vi "HTTPMethod_1.vi"(7 "LabVIEW Web Service Request":refnum<class "Web Request.lvclass">) -> ()   [LabVIEW 2021]
uses:
  <vilib>/wsapi/Web Request.lvclass
panel:
  out "request variables":cluster{"Key":string[], "Value":string[]}
  out "postdata":string
  out "value":string[](array[string])
  # "Use the Web Service Request input terminal to call the VIs on the Web Services palette. Do not remove it from the connector pane unless you don't need access to the palette."
  # "Each additional control wired to the connector pane will be available as an input in the URL. To include an indicator in terminal-mode output (the default setting), it must also be wired to the connector pane."
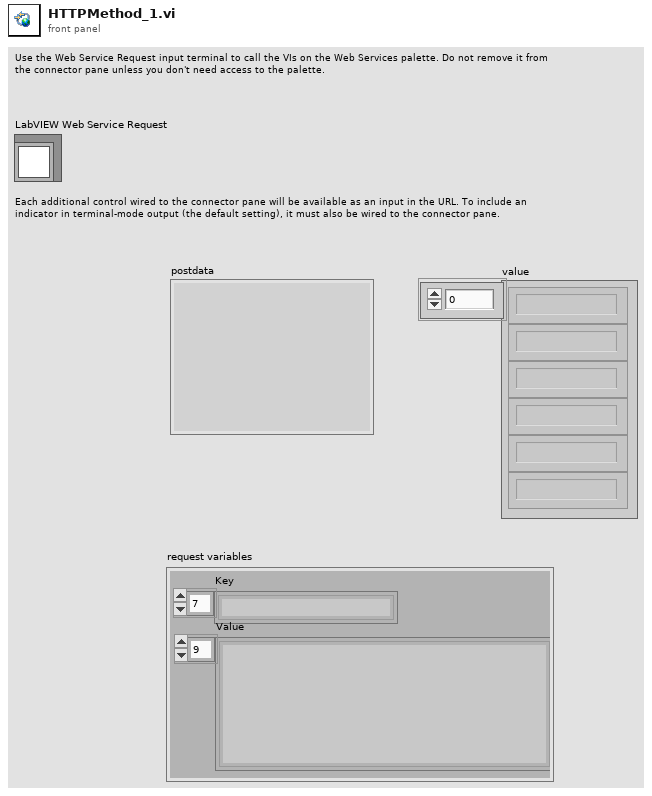
[diagram p1: front panel]
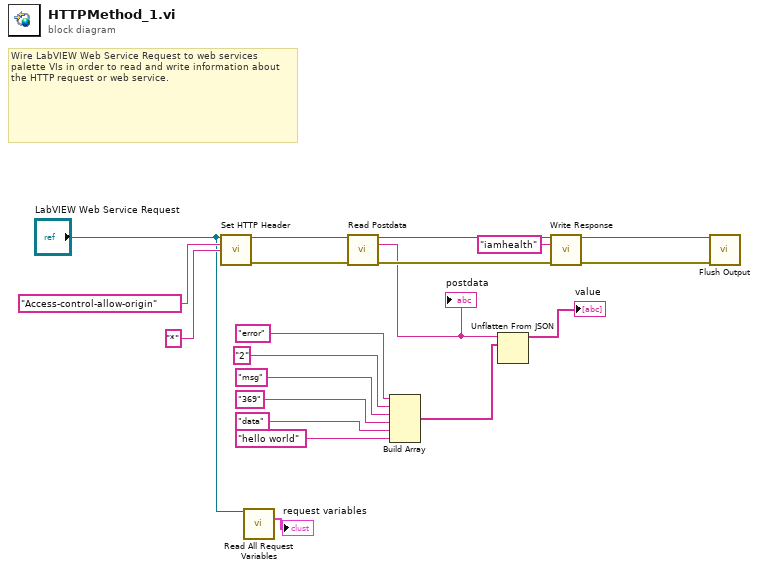
[diagram p0: block diagram]
diagram:
  # "Wire LabVIEW Web Service Request to web services palette VIs in order to read and write information about the HTTP request or web service."
  n1 = call <vilib>:"Set HTTP Header.vi"("LabVIEW Web Service Request"="LabVIEW Web Service Request", "header"="Access-control-allow-origin", "header value"="*") -> ("LabVIEW Web Service Request out"=w20:refnum<class "Web Request.lvclass">, "error out"=w19:errorcluster)  [unwired: 11 in]
  n2 = call <vilib>:"Read All Request Variables.vi"("LabVIEW Web Service Request"="LabVIEW Web Service Request") -> ("request variables"=→"request variables":cluster{"Key":string[], "Value":string[]})  [unwired: 12 in, 2 out]
  n3 = call <vilib>:"Read Postdata.vi"("LabVIEW Web Service Request"=w20, "error in (no error)"=w19) -> ("LabVIEW Web Service Request out"=w18:refnum<class "Web Request.lvclass">, "postdata"=w6:string, "error out"=w17:errorcluster)  [unwired: 11 in]
  "postdata" <- w6
  n4 = Build Array("error", "2", "msg", "369", "data", "hello world") -> (w8:string[])
  n5 = Unflatten From JSON(JSON string=w6, type and defaults=w8) -> (value=→"value":string[])  [unwired: 5 in, 1 out]
  n6 = call <vilib>:"Write Response.vi"("LabVIEW Web Service Request"=w18, "response string"="iamhealth", "error in (no error)"=w17) -> ("LabVIEW Web Service Request out"=w5:refnum<class "Web Request.lvclass">, "error out"=w4:errorcluster)  [unwired: 11 in]
  n7 = call <vilib>:"Flush Output.vi"("LabVIEW Web Service Request"=w5, "error in (no error)"=w4) -> ()  [unwired: 12 in, 2 out]
